vi "just looking.vi"() -> ()   [LabVIEW 2020]
panel:
  in  "Tab Control":enum32{"Page 1", "Page 2"}(tab)
  out "Adjusted 2":waveform(dbl)[](graph)
  out "Adjusted":waveform(dbl)[](graph)
  out "Frequency":dbl[][](graph)
  out "Raw s11 ref":dbl[][](graph)
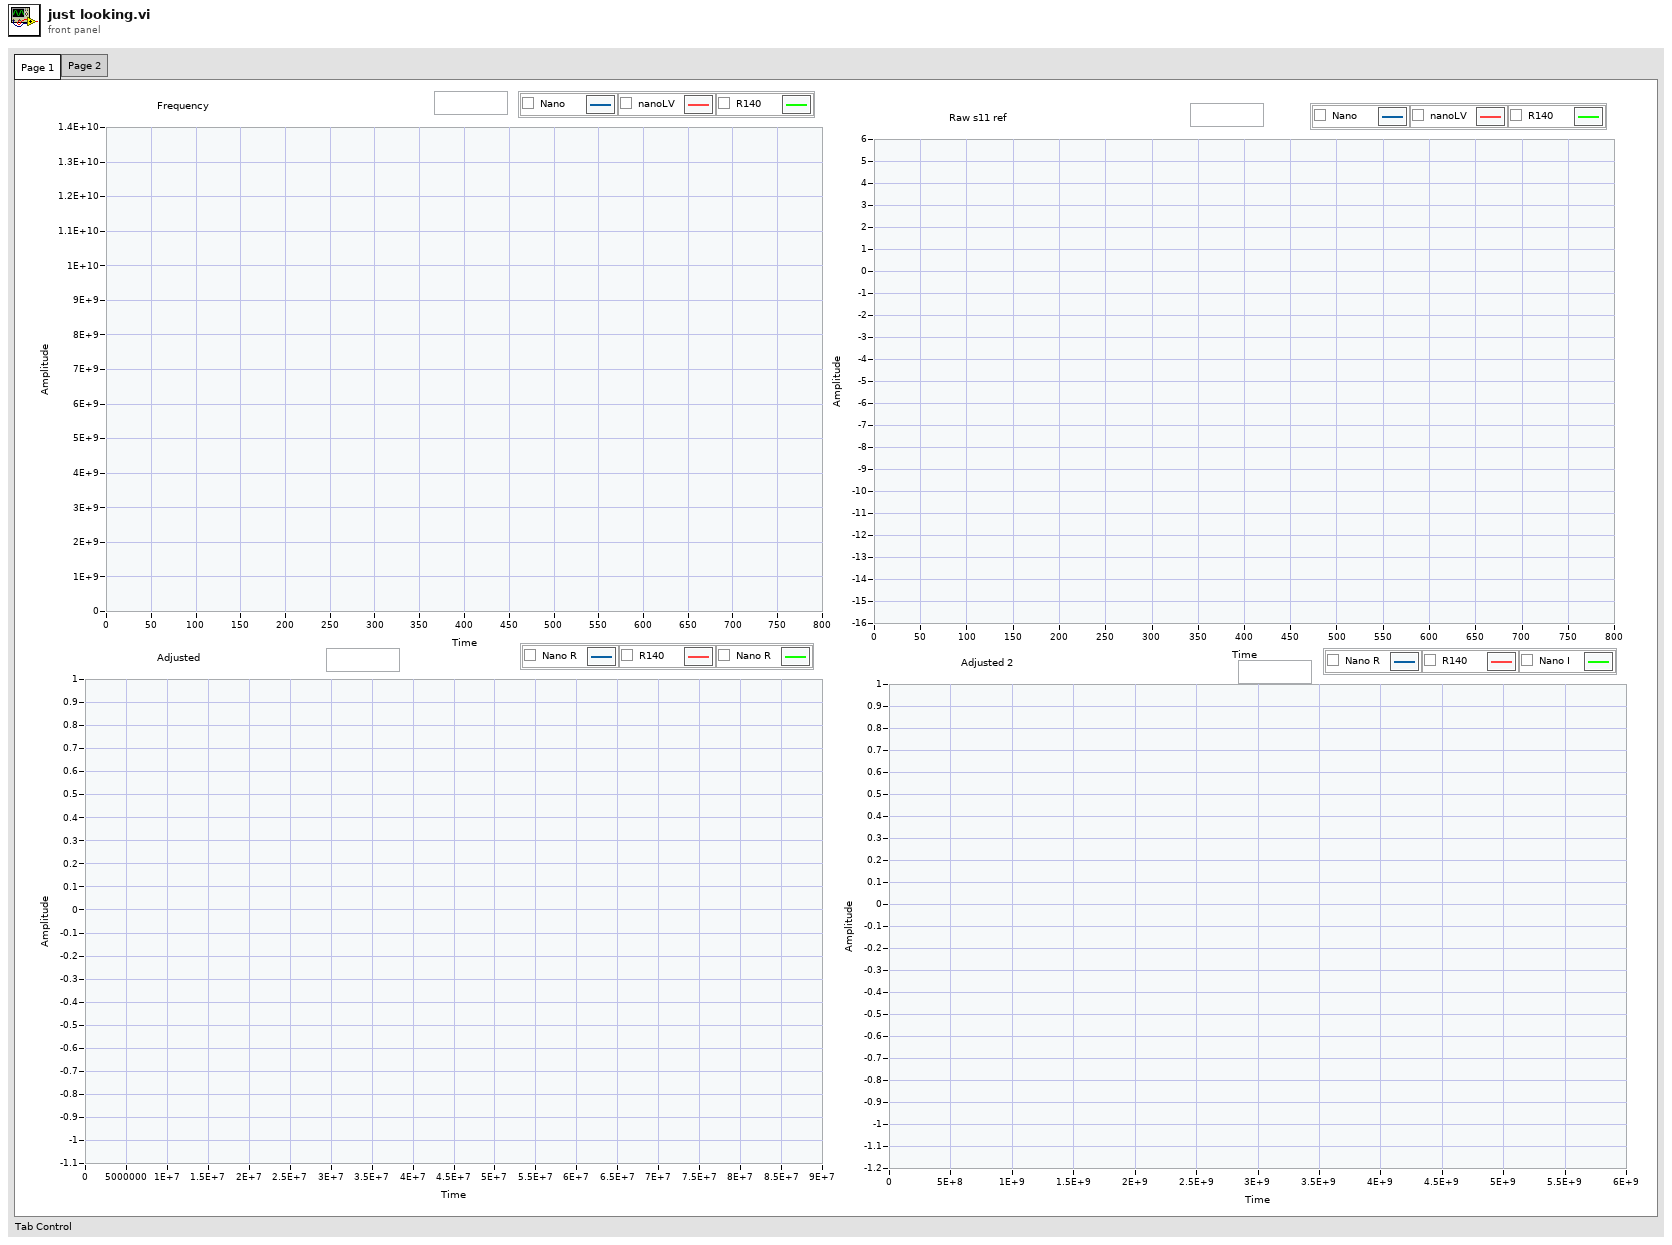
[diagram p1: front panel]
types:
  T1 = typedef "VFH-VNA_File_Handler.lvlib/VFH-file_cluster-Expensive.ctl" = cluster{"Frequency":dbl[], "Permativity'":dbl[], "Permativity''":dbl[], "Q [S/m]":dbl[], "Tan":dbl[], "Reflection R":dbl[], "Reflection I":dbl[]}
  T2 = typedef "VFH-VNA_File_Handler.lvlib/VFH-file_cluster-LabVIEWVNA.ctl" = cluster{"Frequency":dbl[], "S1_Real":dbl[], "S1_Imag":dbl[], "S11_Real":dbl[], "S11_Imag":dbl[], "S21_Real":dbl[], "S21_Imag":dbl[]}
  T3 = typedef "VFH-VNA_File_Handler.lvlib/VFH-file_cluster-NanoVNA.ctl" = cluster{"Frequency":dbl[], "S11_Real":dbl[], "S11_Imag":dbl[], "S21_Real":dbl[], "S21_Imag":dbl[], "S12_Real":dbl[], "S12_Imag":dbl[], "S22_Real":dbl[], "S22_Imag":dbl[]}
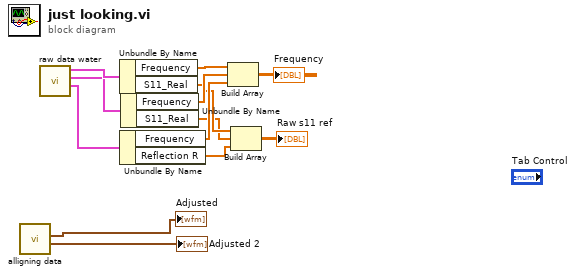
[diagram p0: block diagram]
diagram:
  n1 = call "alligning data.vi"() -> ("Second part"=→"Adjusted 2":waveform(dbl)[], "First Part"=→"Adjusted":waveform(dbl)[])  [unwired: 10 in]
  n2 = call "raw data water.vi"() -> ("output R140"=w11:T1, "avg output LV"=w12:T2, "avg output NV"=w13:T3)  [unwired: 9 in]
  n3 = Unbundle By Name(w13) -> ("Frequency"=w8:dbl[], "S11_Real"=w5:dbl[])
  n4 = Unbundle By Name(w11) -> ("Frequency"=w10:dbl[], "Reflection R"=w3:dbl[])
  n5 = Unbundle By Name(w12) -> ("Frequency"=w9:dbl[], "S11_Real"=w4:dbl[])
  n6 = Build Array(w8, w9, w10) -> (→"Frequency":dbl[][])
  n7 = Build Array(w5, w4, w3) -> (→"Raw s11 ref":dbl[][])
